vi "udc.vi"(11 "Numeric":u8) -> (3 "s? t:f":string)   [LabVIEW 2016]
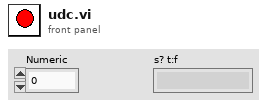
[diagram p1: front panel]
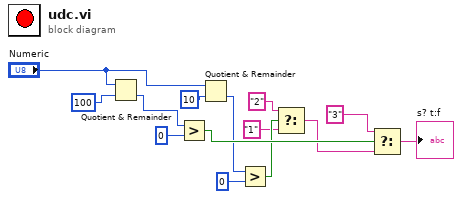
[diagram p0: block diagram]
diagram:
  n1 = Quotient & Remainder(x="Numeric", y=u8 100) -> (floor(x/y)=w12:u8)  [unwired: 1 out]
  n2 = Greater?(x=w12, y=u8 0) -> (0:w10:bool)
  n3 = Quotient & Remainder(x="Numeric", y=u8 10) -> (floor(x/y)=w5:u8)  [unwired: 1 out]
  n4 = Greater?(x=w5, y=u8 0) -> (0:w3:bool)
  n5 = Select(t="2", s=w3, f="1") -> (s? t:f=w7:string)
  n6 = Select(t="3", s=w10, f=w7) -> (s? t:f=→"s? t:f":string)
